vi "test_CCD_Setup_Testenvironment.vi"(8 "error in":errorcluster) -> (0 "error out":errorcluster, 2 "device open for communication?":bool, 3 "CCD out":refnum<class "CCD.lvclass">)   [LabVIEW 2023]
uses:
  Classes/CCD/CCD.lvclass
  Libraries/DeviceManager/DeviceManager.lvlib
panel:
  # "Connector Pane"
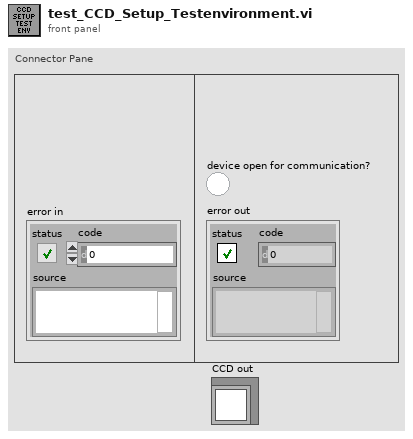
[diagram p1: front panel]
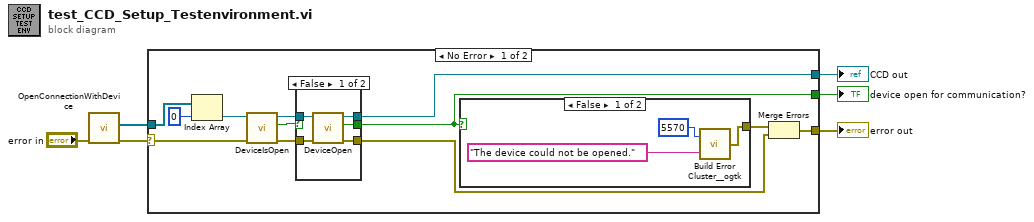
[diagram p0: block diagram]
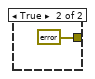
[diagram p3: hidden frame]
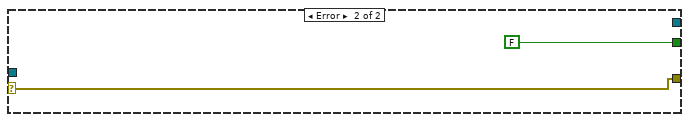
[diagram p4: hidden frame]
diagram:
  n1 = call "OpenConnectionWithDevice.vi"("error in"="error in") -> ("error out"=w1:errorcluster, "CCDs"=w2:refnum<class "CCD.lvclass">[])  [unwired: 7 in, 2 out]
  n2 = case shown="No Error" w1 {
    selector: w1 -> [w8 w32]
    tunnel: w2 -> [w18 _]
    tunnel: [w16 w32] -> w5
    tunnel: [w9 FALSE ("CCD open for communication?")] -> w4
    tunnel: [w10 _] -> w3
    frame No Error {
      n3 = Index Array(array=w18, index=0) -> (element=w11:refnum<class "CCD.lvclass">)
      n4 = call-dynamic "DeviceIsOpen.vi"("error in (no error)"=w8, "CCD in"=w11) -> ("error out"=w12:errorcluster, "device is open?"=w13:bool, "CCD out"=w14:refnum<class "CCD.lvclass">)  [unwired: 6 in, 1 out]
      n5 = case shown="False" w13 {
        selector: w13 -> [_ w24]
        tunnel: [w23 w24] -> w9
        tunnel: [w22 w25] -> w7
        tunnel: [w21 w26] -> w10
        tunnel: w12 -> [w20 w25]
        tunnel: w14 -> [w19 w26]
        frame False {
          n6 = call-dynamic "DeviceOpen.vi"("error in (no error)"=w20, "CCD in"=w19) -> ("error out"=w22:errorcluster, "device is open?"=w23:bool, "CCD out"=w21:refnum<class "CCD.lvclass">)  [unwired: 6 in, 1 out]
        }
        frame True {
        }
      }
      n7 = case shown="False" w9 {
        tunnel: [w28 errorcluster {"status"=FALSE, "code"=0, "source"=""} ("error in 2")] -> w15
        frame False {
          n8 = call <userlib>:"Build Error Cluster__ogtk.vi"("String to Prepend to source (\"\")"="The device could not be opened." ("String to Prepend to source (\"\")"), "code"=5570) -> ("error out"=w28:errorcluster)
        }
        frame True {
        }
      }
      n9 = Merge Errors(w15, w7) -> (w16:errorcluster)
    }
    frame Error {
    }
  }
  "error out" <- w5
  "device open for communication?" <- w4
  "CCD out" <- w3
